vi "Scan Engine Custom Main IO Network Variables.vi"(8 "error in (no error)":errorcluster, 11 "Node Ptr":T1 format="%.0x") -> (0 "error out":errorcluster)   [LabVIEW 2020, in "SEECD System Explorer.lvlib"]
uses:
  SEECD System Explorer.lvlib
  <vilib>/NI VeriStand/Custom Device API/Custom Device Item Ref.ctl
  <vilib>/NI VeriStand/Custom Device API/Custom Device API.lvlib
panel:
  in  "SHDocVw.IWebBrowser2":refnum<k7>(container)
  in  "Header":cluster{"Section Name":string}={"Section Name"=" I/O Network Variables Section"}
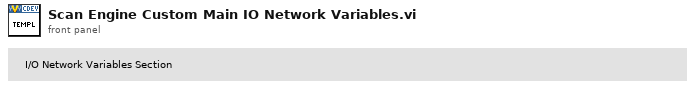
[diagram p1: front panel]
types:
  T1 = typedef "Custom Device API.lvlib/Custom Device Item Ref.ctl" = u64
  T2 = typedef "Custom Device API.lvlib/Custom Device Commands.ctl" = enum16{"Default", "Item renamed", "Shutdown", "Dynamic button pressed"}
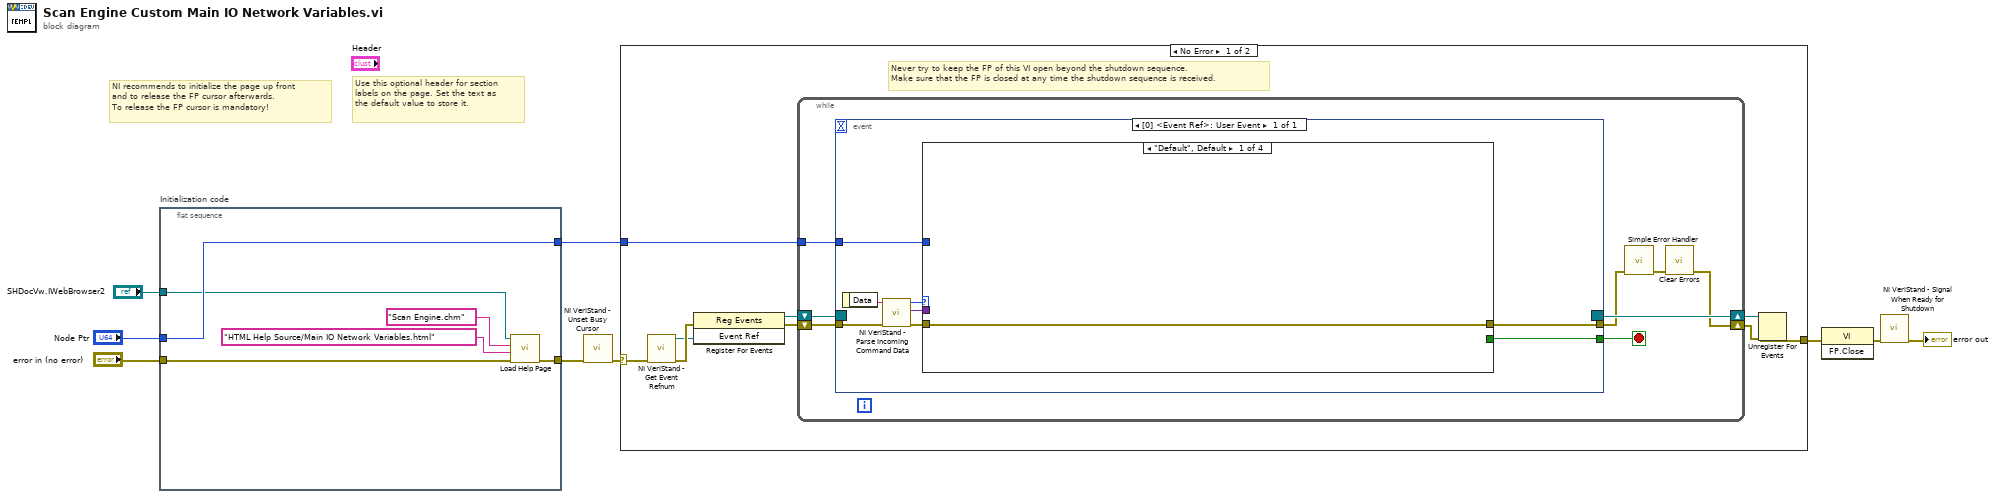
[diagram p0: block diagram]
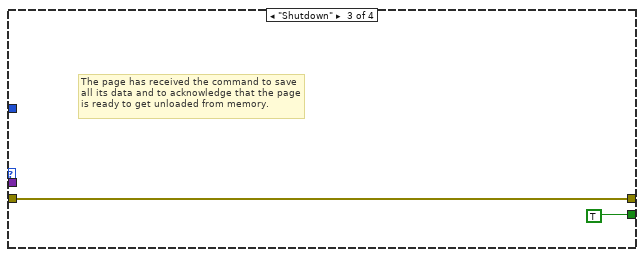
[diagram p3: hidden frame]
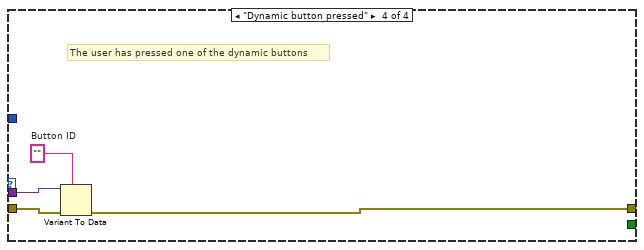
[diagram p4: hidden frame]
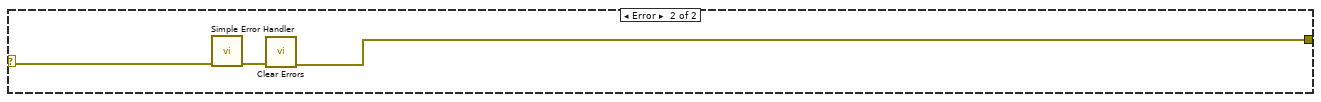
[diagram p5: hidden frame]
diagram:
  # "Use this optional header for section labels on the page. Set the text as the default value to store it."
  # "NI recommends to initialize the page up front\nand to release the FP cursor afterwards.\nTo release the FP cursor is mandatory!"
  n1 = flat-sequence "Initialization code" {
    tunnel: "error in (no error)" -> [w12]
    tunnel: "Node Ptr" -> [w15]
    tunnel: [w11] -> w5
    tunnel: [w15] -> w2
    tunnel: "SHDocVw.IWebBrowser2" -> [w10]
    frame #0 {
      n2 = call "Load Help Page.vi"("error in (no error)"=w12, "HTML File to Load"="HTML Help Source/Main IO Network Variables.html" ("name or relative path"), "Main CHM File"="Scan Engine.chm" ("name or relative path"), "Browser"=w10) -> ("error out"=w11:errorcluster)  [unwired: 7 in]
    }
  }
  n3 = call <vilib>:"NI VeriStand - Unset Busy Cursor.vi"("error in (no error)"=w5) -> ("error out"=w4:errorcluster)  [unwired: 10 out]
  n4 = case shown="No Error" w4 {
    selector: w4 -> [w16 w51]
    tunnel: [w21 w49] -> w9
    tunnel: w2 -> [w17 _]
    frame No Error {
      # "Never try to keep the FP of this VI open beyond the shutdown sequence.\nMake sure that the FP is closed at any time the shutdown sequence is received."
      n5 = call <vilib>:"NI VeriStand - Get Event Refnum.vi"("error in (no error)"=w16) -> ("error out"=w24:errorcluster, "Event Ref"=w20:refnum<user-event>)  [unwired: 9 out]
      n6 = register-events(error in=w24, w20) -> (reference out=w18:refnum<event-registration>, error out=w19:errorcluster)  [unwired: 1 in]
      n7 = while {
        tunnel: w17 -> [w28]
        shift-right: [w25] -> w22
        shift-left: w19 -> [w31]
        shift-right: [w32] -> w23
        shift-left: w18 -> [w30]
        stop <- w29 stop-if-true
        n8 = event shown="[0] <Event Ref>: User Event" {
          selector: w30 -> [_]
          dyn-events: [_] -> w32
          timeout: _ -> [_]
          tunnel: w31 -> [w40]
          tunnel: [w36] -> w29
          tunnel: [w35] -> w27
          tunnel: w28 -> [w34]
          event User Event {
            n9 = event-data() -> ("Data"=w39:string)  [unwired: 1 out]
            n10 = call <vilib>:"NI VeriStand - Parse Incoming Command Data.vi"("error in (no error)"=w40, "Incoming data"=w39) -> ("error out"=w38:errorcluster, "Outgoing data"=w33:variant, "Action"=w37:T2)  [unwired: 7 out]
            n11 = case shown="\"Default\", Default" w37 {
              tunnel: w38 -> [w41 w42 w43 w48]
              tunnel: [_ _ TRUE _] -> w36
              tunnel: [w41 w42 w43 w45] -> w35
              tunnel: w34 -> [_ _ _ _]
              tunnel: w33 -> [_ _ _ w47]
              frame "Default", Default {
              }
              frame "Item renamed" {
              }
              frame "Shutdown" {
                # "The page has received the command to save all its data and to acknowledge that the page is ready to get unloaded from memory."
              }
              frame "Dynamic button pressed" {
                w46 = ""  # Button ID
                # "The user has pressed one of the dynamic buttons"
                n12 = Variant To Data(error in=w48, type=w46, Variant=w47) -> (error out=w45:errorcluster)  [unwired: 1 out]
              }
            }
          }
        }
        n13 = call <vilib>:"Simple Error Handler.vi"("error in (no error)"=w27) -> ("error out"=w26:errorcluster)  [unwired: 1 in, 7 out]
        n14 = call <vilib>:"Clear Errors.vi"("error in (no error)"=w26) -> ("error out"=w25:errorcluster)  [unwired: 1 in, 5 out]
      }
      n15 = Unregister For Events(event registration refnum=w23, error in=w22) -> (error out=w21:errorcluster)
    }
    frame Error {
      n16 = call <vilib>:"Simple Error Handler.vi"("error in (no error)"=w51) -> ("error out"=w50:errorcluster)  [unwired: 1 in, 7 out]
      n17 = call <vilib>:"Clear Errors.vi"("error in (no error)"=w50) -> ("error out"=w49:errorcluster)  [unwired: 1 in, 5 out]
    }
  }
  n18 = invoke class="VI" method="FP.Close"(error in=w9) -> (error out=w8:errorcluster)  [unwired: 2 in, 2 out]
  n19 = call <vilib>:"NI VeriStand - Signal When Ready for Shutdown.vi"("error in (no error)"=w8) -> ("error out"=→"error out":errorcluster)  [unwired: 10 out]
